vi "Initialize Module.vi"(8 "error in (no error)":errorcluster) -> (0 "error out":errorcluster)   [LabVIEW 2023, in "Template.lvlib"]
doc: "VI used to initialize module, create queue and events."
uses:
  Template.lvlib
  Type Def/Message Data.ctl
  Type Def/FGV Queue State.ctl
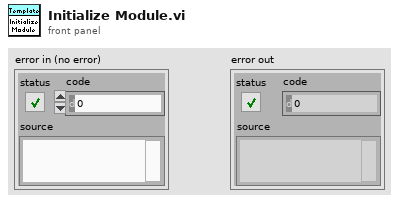
[diagram p1: front panel]
types:
  T1 = typedef "Template.lvlib/FGV Queue State.ctl" = enum16{"Get", "Set"}
  T2 = typedef "Template.lvlib/Message Data.ctl" = cluster{"Message":string, "Data":variant}
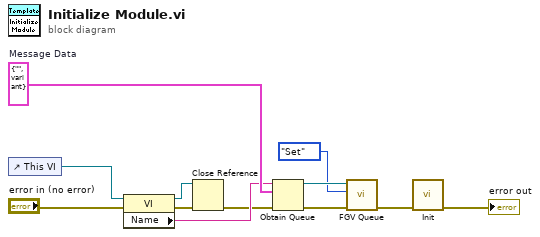
[diagram p0: block diagram]
diagram:
  w12 = T2 {"Message"="", "Data"=variant}  # Message Data
  n1 = control-ref of="This VI"() -> (w10:refnum<vi>)
  n2 = property class="VI"(reference=w10, error in="error in (no error)") -> (reference out=w8:refnum<vi>, error out=w9:errorcluster, "Name"=w7:string)
  n3 = Close Reference(reference=w8, error in (no error)=w9) -> (error out=w6:errorcluster)
  n4 = Obtain Queue(name (unnamed)=w7, element data type=w12, error in (no error)=w6) -> (queue out=w4:refnum<queue>, error out=w2:errorcluster)  [unwired: 2 in, 1 out]
  n5 = call "FGV Queue.vi"("error in (no error)"=w2, "FGV Queue State"=FGV_Queue_State."Set", "queue in"=w4) -> ("error out"=w1:errorcluster)  [unwired: 7 in, 1 out]
  n6 = call "Init.vi"("error in (no error)"=w1) -> ("error out"=→"error out":errorcluster)  [unwired: 10 in]
